vi "Test Data Logger v2 API.vi"() -> ()   [LabVIEW 2025, in "Data Logger v2.lvlib"]
doc: "Data Logger v2 API Tester.\n\n<b>Note:</b> This VI was modified by the <b>Validate DQMH Module</b> tool to upgrade it to the DQMH 5.0 approach to only call the Stop Module.vi at the end of the tester if the module wasn't originally running when the tester started.\n\n<b>Note:</b> This VI was modified by the <b>Validate DQMH Module</b> tool to upgrade its Error Reported event frame to use an improved mechanism for displaying error information.\n\n<b>Note:</b> This VI was modified by the <b>Validate DQMH Module</b> tool to remove code to stop the main loop on error, and instead display the most recent error on the tester front panel."
uses:
  Data Logger v2.lvlib
  Write TDMS 2D Array Parameters--cluster.ctl
  Write TDMS 2D String Array Parameters--cluster.ctl
  <vilib>/Utility/error.llb/DialogType.ctl
  <vilib>/MGI/Panel Manager/Panel/Panel/Window/Window.lvclass
  <vilib>/MGI/Panel Manager/Panel/Panel/Window/Dialog/Dialog.lvclass
  <vilib>/MGI/Panel Manager/Panel/Panel/Subpanel/Subpanel.lvclass
  <vilib>/MGI/Panel Manager/Panel/Panel/Window/Window.vi
  <vilib>/MGI/Panel Manager/Panel/Panel/Window/Dialog/Dialog.vi
  <vilib>/MGI/Panel Manager/Panel/Panel/Subpanel/Subpanel.vi
  <vilib>/MGI/Panel Manager/Panel/Panel.lvlib
panel:
  in  "Property names":string[](array[string])
  in  "Property values":variant[](array[variant])
  in  "Group name":string
  in  "Channel name":string
  in  "Set Properties":bool
  out "last error":errorcluster
  in  "Filename":string
  in  "Create New TDMS Log File (Relative Path)":bool
  in  "Root Folder Path":path
  in  "Set Root Folder Path":bool
  in  "TDMS Write 2D String Array Parameters":T1
  in  "Write TDMS 2D String Array":bool
  in  "Close TDMS File":bool
  in  "TDMS Write 2D Array Parameters":T2
  in  "Write 2D Array to TDMS Log File":bool
  in  "File Path (inc. Filename)":path
  in  "Create New TDMS Log File":bool
  in  "Autoshow?":bool
  in  "Panel Type":enum16{"Window", "Dialog", "Subpanel"}(ring)
  in  "Change Panel":bool
  in  "Tab Control":enum32{"Status", "Subpanel"}(tab)
  out "Status":string
  in  "Show Block Diagram":bool
  in  "Stop Module":bool
  in  "Start Module":bool
  in  "Hide Module Panel":bool
  in  "Show Module Panel":bool
  out "Module Running?":bool
  # "This VI tests the API for the Module."
  # "Change Panel"
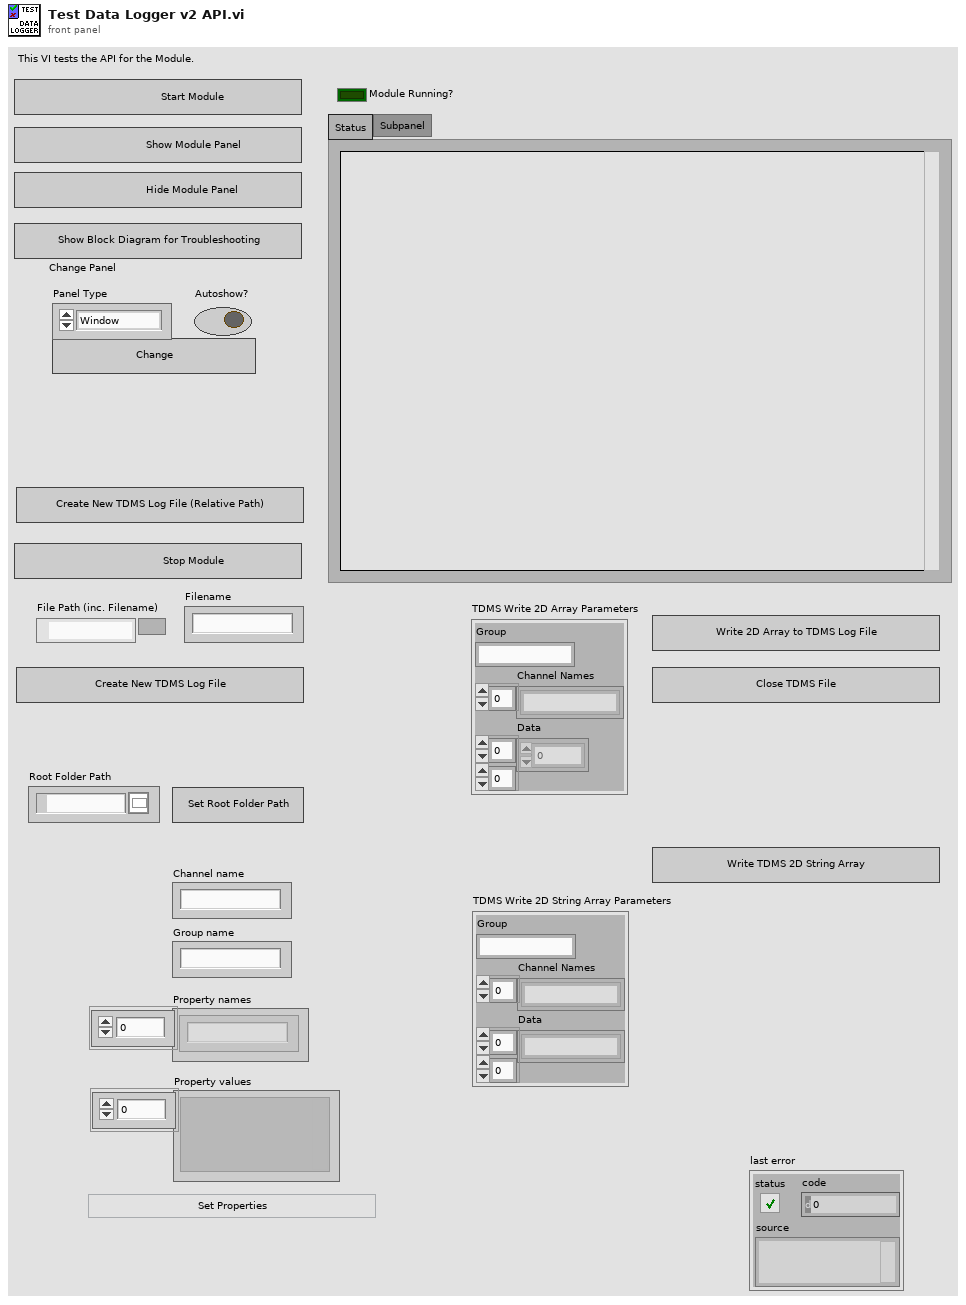
[diagram p1: front panel]
types:
  T1 = typedef "Data Logger v2.lvlib/Write TDMS 2D String Array Parameters--cluster.ctl" = cluster{"Group":string, "Channel Names":string[], "Data":string[][]}
  T2 = typedef "Data Logger v2.lvlib/Write TDMS 2D Array Parameters--cluster.ctl" = cluster{"Group":string, "Channel Names":string[], "Data":dbl[][]}
  T3 = typedef "Data Logger v2.lvlib/Broadcast Events--cluster.ctl" = cluster{"Module Did Init":refnum<user-event>, "Status Updated":refnum<user-event>, "Error Reported":refnum<user-event>, "Module Did Stop":refnum<user-event>, "Update Module Execution Status":refnum<user-event>}
  T4 = typedef "DialogType.ctl" = u16
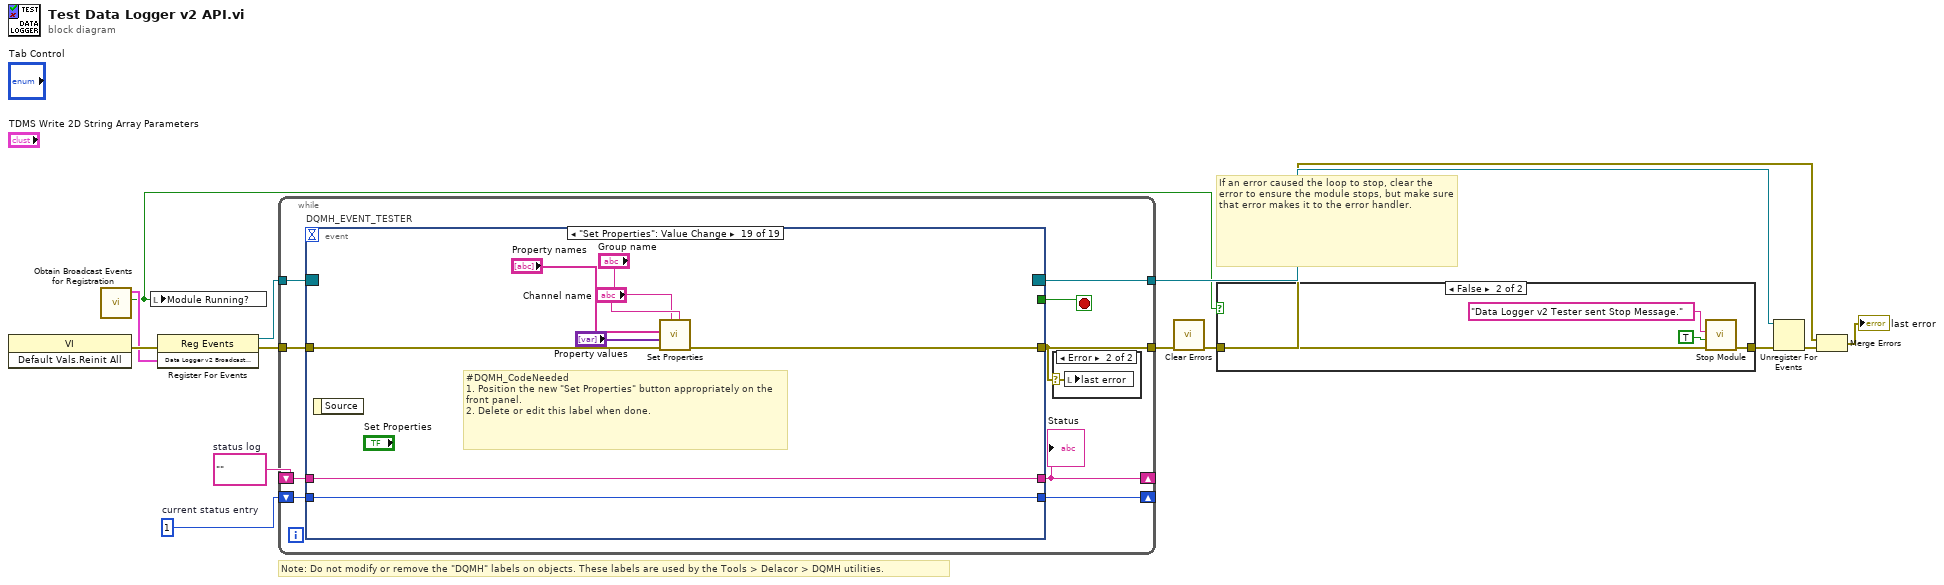
[diagram p0: block diagram]
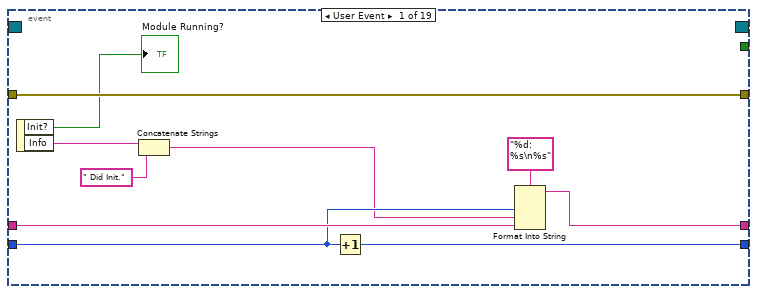
[diagram p4: hidden frame]
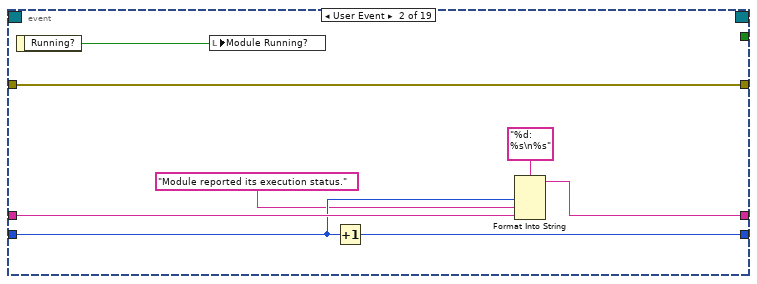
[diagram p5: hidden frame]
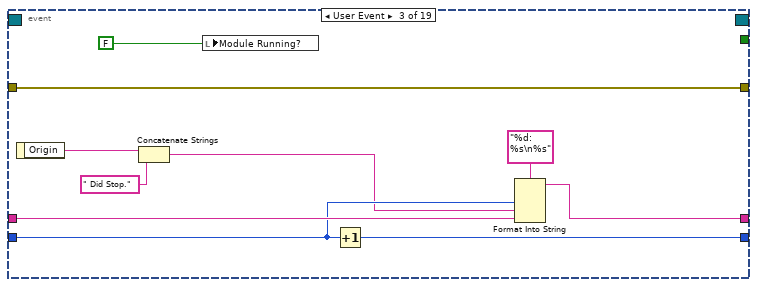
[diagram p6: hidden frame]
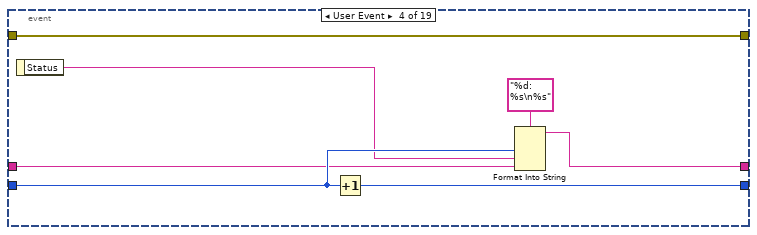
[diagram p7: hidden frame]
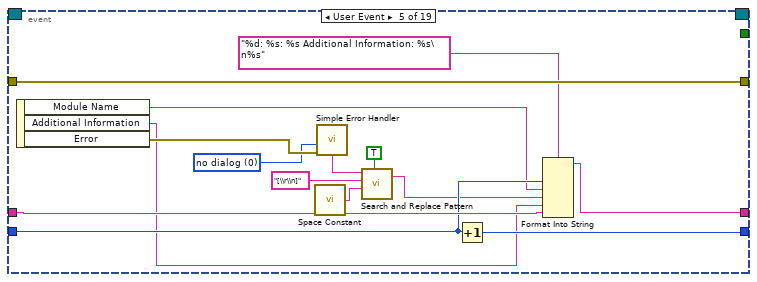
[diagram p8: hidden frame]
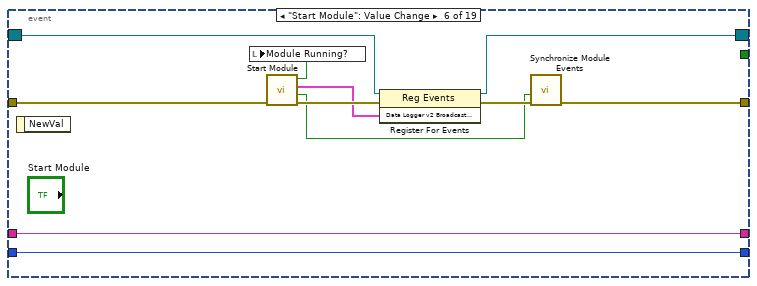
[diagram p9: hidden frame]
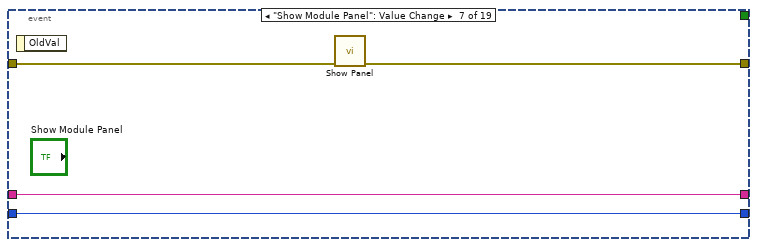
[diagram p10: hidden frame]
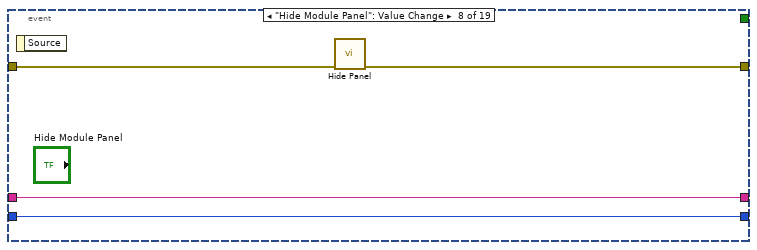
[diagram p11: hidden frame]
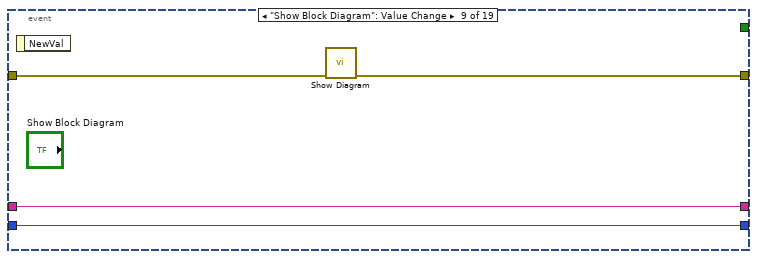
[diagram p12: hidden frame]
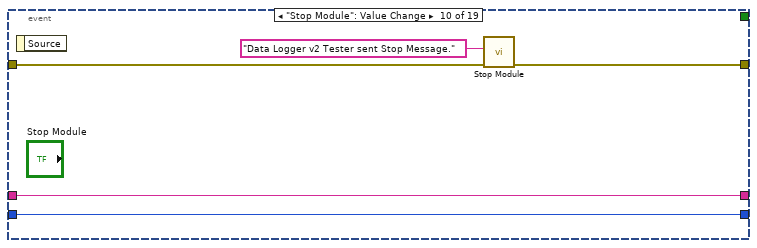
[diagram p13: hidden frame]
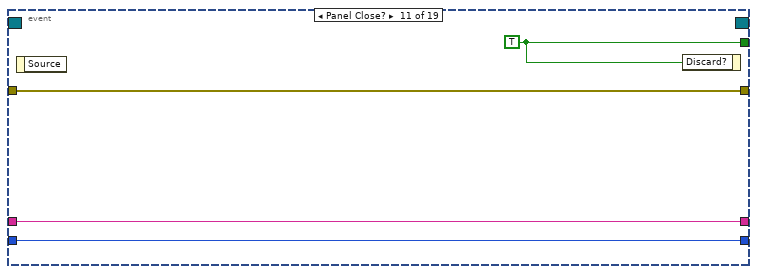
[diagram p14: hidden frame]
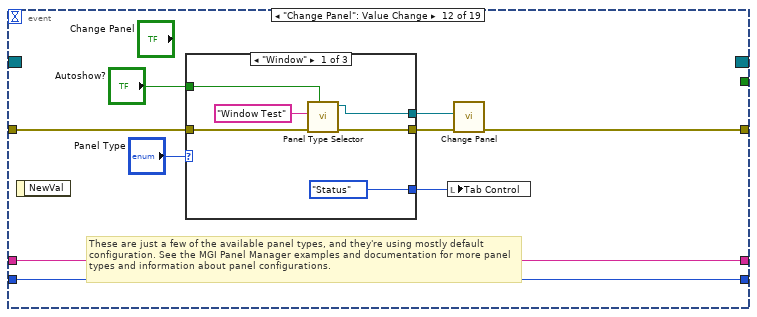
[diagram p15: hidden frame]
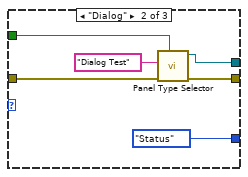
[diagram p16: hidden frame]
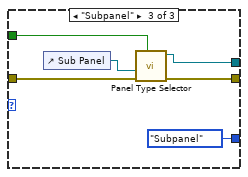
[diagram p17: hidden frame]
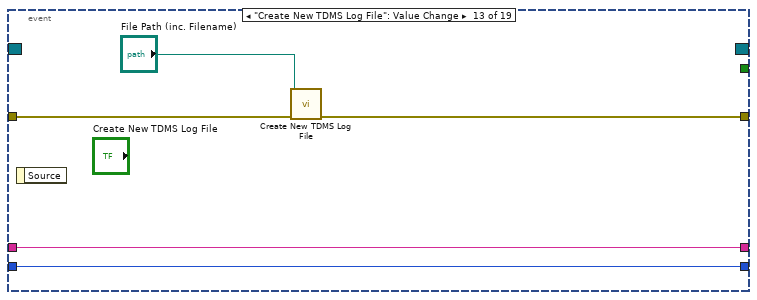
[diagram p18: hidden frame]
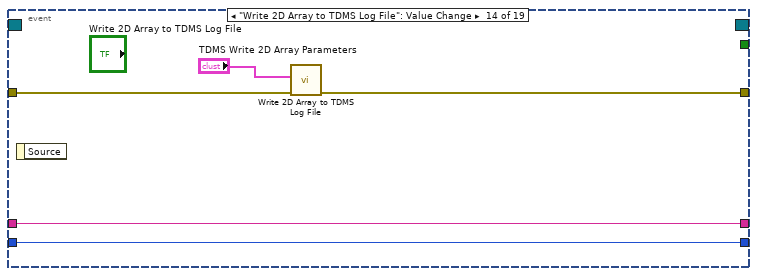
[diagram p19: hidden frame]
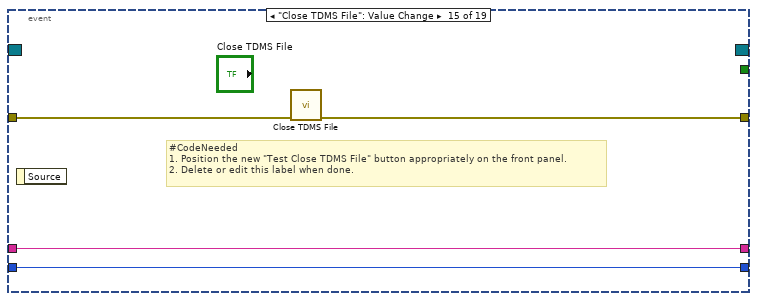
[diagram p20: hidden frame]
diagram:
  w10 = 1  # current status entry
  w11 = ""  # status log
  # "If an error caused the loop to stop, clear the error to ensure the module stops, but make sure that error makes it to the error handler."
  # "Note: Do not modify or remove the \"DQMH\" labels on objects. These labels are used by the Tools > Delacor > DQMH utilities."
  n1 = invoke class="VI" method="Default Vals.Reinit All"() -> (error out=w9:errorcluster)  [unwired: 3 in, 2 out]
  n2 = call "Obtain Broadcast Events for Registration.vi"() -> ("Already running?"=w2:bool, "Data Logger v2 Broadcast Events"=w7:T3)  [unwired: 9 in, 1 out]
  n3 = local write "Module Running?"(w2) -> ()
  n4 = register-events(error in=w9, w7) -> (reference out=w6:refnum<event-registration>, error out=w8:errorcluster)  [unwired: 1 in]
  n5 = while {
    tunnel: w6 -> [w22]
    tunnel: [w15] -> w3
    shift-right: [w18] -> _
    shift-left: w11 -> [w20]
    shift-right: [w19] -> _
    shift-left: w10 -> [w21]
    tunnel: w8 -> [w17]
    tunnel: [w16] -> w5
    stop <- w14 stop-if-true
    n6 = event "DQMH_EVENT_TESTER" shown="[18] \"Set Properties\": Value Change" {
      selector: w22 -> [_ _ _ _ _ w78 _ _ _ _ _ _ _ _ _ _ _ _ _]
      dyn-events: [_ _ _ _ _ w77 _ _ _ _ _ _ _ _ _ _ _ _ _] -> w16
      timeout: _ -> [_ _ _ _ _ _ _ _ _ _ _ _ _ _ _ _ _ _ _]
      tunnel: [_ _ _ _ _ _ _ _ _ _ w105 _ _ _ _ _ _ _ _] -> w14
      tunnel: [w33 w35 w42 w52 w73 w76 w88 w92 w93 w99 w102 w112 w134 w139 w143 w147 w152 w157 w165] -> w15
      tunnel: w21 -> [w29 w39 w49 w55 w70 w81 w86 w90 w94 w100 w103 w113 w135 w140 w144 w148 w153 w158 w166]
      tunnel: w20 -> [w30 w40 w50 w54 w72 w82 w87 w91 w95 w101 w104 w114 w136 w141 w145 w149 w154 w159 w167]
      tunnel: [w27 w37 w47 w56 w71 w82 w87 w91 w95 w101 w104 w114 w136 w141 w145 w149 w154 w159 w167] -> w18
      tunnel: [w28 w38 w48 w58 w69 w81 w86 w90 w94 w100 w103 w113 w135 w140 w144 w148 w153 w158 w166] -> w19
      tunnel: w17 -> [w33 w35 w42 w52 w73 w74 w85 w89 w96 w97 w102 w111 w137 w142 w146 w150 w155 w160 w168]
      event User Event {
        n7 = event-data() -> ("Init?"=→"Module Running?":bool, "Info"=w26:string)  [unwired: 1 in]
        n8 = Concatenate Strings(w26, " Did Init.") -> (w25:string)
        n9 = Increment(x=w29) -> (x+1=w28:i32)
        n10 = Format Into String(format string="%d: %s\n%s", w29, w25, w30) -> (resulting string=w27:string)  [unwired: 2 in, 1 out]
      }
      event User Event {
        n11 = event-data() -> ("Running?"=w34:bool)  [unwired: 1 in]
        n12 = local write "Module Running?"(w34) -> ()
        n13 = Increment(x=w39) -> (x+1=w38:i32)
        n14 = Format Into String(format string="%d: %s\n%s", w39, "Module reported its execution status.", w40) -> (resulting string=w37:string)  [unwired: 2 in, 1 out]
      }
      event User Event {
        n15 = event-data() -> ("Origin"=w46:string)  [unwired: 1 in]
        n16 = Concatenate Strings(w46, " Did Stop.") -> (w45:string)
        n17 = local write "Module Running?"(FALSE ("Module Did Init?")) -> ()
        n18 = Increment(x=w49) -> (x+1=w48:i32)
        n19 = Format Into String(format string="%d: %s\n%s", w49, w45, w50) -> (resulting string=w47:string)  [unwired: 2 in, 1 out]
      }
      event User Event {
        n20 = event-data() -> ("Status"=w53:string)  [unwired: 1 in]
        n21 = Increment(x=w55) -> (x+1=w58:i32)
        n22 = Format Into String(format string="%d: %s\n%s", w55, w53, w54) -> (resulting string=w56:string)  [unwired: 2 in, 1 out]
      }
      event User Event {
        w65 = T4 0 items=["no dialog", "OK message", "continue or stop message", "OK message + warnings", "continue/stop + warnings"] ("type of dialog (OK msg:1)")
        n23 = event-data() -> ("Module Name"=w66:string, "Additional Information"=w67:string, "Error"=w68:errorcluster)  [unwired: 1 in]
        n24 = call <vilib>:"Space Constant.vi"() -> ("String"=w61:string)
        n25 = call <vilib>:"Simple Error Handler.vi"("type of dialog (OK msg:1)"=w65, "error in (no error)"=w68) -> ("message"=w64:string)  [unwired: 3 in, 4 out]
        n26 = call <vilib>:"Search and Replace Pattern.vi"("string"=w64, "regular expression (\"\")"="[\\r\\n]" ("regular expression (\"\")"), "replace string (\"\")"=w61, "replace all? (F)"=TRUE ("replace all CR/LF with spaces")) -> ("result string"=w63:string)  [unwired: 1 in, 1 out]
        n27 = Increment(x=w70) -> (x+1=w69:i32)
        n28 = Format Into String(format string="%d: %s: %s Additional Information: %s\n%s", w70, w66, w63, w67, w72) -> (resulting string=w71:string)  [unwired: 2 in, 1 out]
      }
      event "Start Module": Value Change {
        n29 = event-data() -> ()  [unwired: 1 in, 1 out]
        n30 = call "Start Module.vi"("error in (no error)"=w74) -> ("error out"=w83:errorcluster, "Wait for Event Sync?"=w80:bool, "Data Logger v2 Broadcast Events"=w79:T3, "Module Was Already Running?"=w75:bool)  [unwired: 7 in]
        n31 = local write "Module Running?"(w75) -> ()
        n32 = register-events(reference=w78, error in=w83, w79) -> (reference out=w77:refnum<event-registration>, error out=w84:errorcluster)
        n33 = call "Synchronize Module Events.vi"("error in (no error)"=w84, "Wait for Event Sync?"=w80) -> ("error out"=w76:errorcluster)  [unwired: 9 in]
      }
      event "Show Module Panel": Value Change {
        n34 = event-data() -> ()  [unwired: 1 in, 1 out]
        n35 = call "Show Panel.vi"("error in (no error)"=w85) -> ("error out"=w88:errorcluster)  [unwired: 10 in]
      }
      event "Hide Module Panel": Value Change {
        n36 = event-data() -> ()  [unwired: 1 in, 1 out]
        n37 = call "Hide Panel.vi"("error in (no error)"=w89) -> ("error out"=w92:errorcluster)  [unwired: 10 in]
      }
      event "Show Block Diagram": Value Change {
        n38 = event-data() -> ()  [unwired: 1 in, 1 out]
        n39 = call "Show Diagram.vi"("error in (no error)"=w96) -> ("error out"=w93:errorcluster)  [unwired: 10 in]
      }
      event "Stop Module": Value Change {
        n40 = event-data() -> ()  [unwired: 1 in, 1 out]
        n41 = call "Stop Module.vi"("error in (no error)"=w97, "Origin"="Data Logger v2 Tester sent Stop Message.") -> ("error out"=w99:errorcluster)  [unwired: 9 in]
      }
      event Panel Close? {
        w105 = TRUE ("Discard?")
        n42 = event-data() -> ()  [unwired: 1 in, 1 out]
        n43 = event-data("Discard?"=w105) -> ()  [unwired: 1 in, 1 out]
      }
      event "Change Panel": Value Change {
        # "These are just a few of the available panel types, and they're using mostly default configuration. See the MGI Panel Manager examples and documentation for more panel types and information about panel configurations."
        n44 = event-data() -> ()  [unwired: 1 in, 1 out]
        n45 = case shown="\"Window\"" "Panel Type" {
          tunnel: w111 -> [w120 w126 w132]
          tunnel: [w119 w125 w131] -> w110
          tunnel: [w118 w124 w130] -> w109
          tunnel: [enum32{"Status", "Subpanel"}."Status" ("Tab Control") enum32{"Status", "Subpanel"}."Status" ("Tab Control") enum32{"Status", "Subpanel"}."Subpanel" ("Tab Control")] -> w107
          tunnel: "Autoshow?" -> [w115 w121 w127]
          frame "Window" {
            n46 = call-poly <vilib>:"Panel Type Selector.vi"("Autoshow? (T)"=w115, "error in (no error)"=w120, "Default Title"="Window Test") -> ("error out"=w119:errorcluster, "Window out"=w118:refnum<class "Window.lvclass">)  [unwired: 7 in]
          }
          frame "Dialog" {
            n47 = call-poly <vilib>:"Panel Type Selector.vi"("Autoshow? (T)"=w121, "Error In"=w126, "Default Title"="Dialog Test") -> ("Error Out"=w125:errorcluster, "Dialog out"=w124:refnum<class "Dialog.lvclass">)  [unwired: 7 in]
          }
          frame "Subpanel" {
            n48 = control-ref of="Sub Panel"() -> (w129:refnum<vi>)
            n49 = call-poly <vilib>:"Panel Type Selector.vi"("Autoshow? (T)"=w127, "Error In"=w132, "Sub Panel"=w129) -> ("Error Out"=w131:errorcluster, "Subpanel Out"=w130:refnum<class "Subpanel.lvclass">)  [unwired: 7 in]
          }
        }
        n50 = local write "Tab Control"(w107) -> ()
        n51 = call "Change Panel.vi"("error in (no error)"=w110, "New Panel"=w109) -> ("error out"=w112:errorcluster)  [unwired: 9 in]
      }
      event "Create New TDMS Log File": Value Change {
        n52 = event-data() -> ()  [unwired: 1 in, 1 out]
        n53 = call "Create New TDMS Log File.vi"("error in (no error)"=w137, "File Path (inc. Filename)"="File Path (inc. Filename)") -> ("error out"=w134:errorcluster)  [unwired: 9 in]
      }
      event "Write 2D Array to TDMS Log File": Value Change {
        n54 = event-data() -> ()  [unwired: 1 in, 1 out]
        n55 = call "Write 2D Array to TDMS Log File.vi"("error in (no error)"=w142, "TDMS Write 2D Array Parameters"="TDMS Write 2D Array Parameters") -> ("error out"=w139:errorcluster)  [unwired: 9 in]
      }
      event "Close TDMS File": Value Change {
        # "#CodeNeeded\n1. Position the new \"Test Close TDMS File\" button appropriately on the front panel.\n2. Delete or edit this label when done."
        n56 = event-data() -> ()  [unwired: 1 in, 1 out]
        n57 = call "Close TDMS File.vi"("error in (no error)"=w146) -> ("error out"=w143:errorcluster)  [unwired: 10 in]
      }
      event "Write TDMS 2D String Array": Value Change {
        # "#CodeNeeded\n1. Position the new \"Test Write TDMS 2D String Array\" button appropriately on the front panel.\n2. Delete or edit this label when done."
        n58 = event-data() -> ()  [unwired: 1 in, 1 out]
        n59 = call "Write TDMS 2D String Array.vi"("error in (no error)"=w150) -> ("error out"=w147:errorcluster)  [unwired: 10 in]
      }
      event "Set Root Folder Path": Value Change {
        # "#CodeNeeded\n1. Position the new \"Test Set Root Folder Path\" button appropriately on the front panel.\n2. Delete or edit this label when done."
        n60 = event-data() -> ()  [unwired: 1 in, 1 out]
        n61 = call "Set Root Folder Path.vi"("error in (no error)"=w155, "Root Folder Path"="Root Folder Path") -> ("error out"=w152:errorcluster)  [unwired: 9 in]
      }
      event "Create New TDMS Log File (Relative Path)": Value Change {
        # "#CodeNeeded\n1. Position the new \"Test Create New TDMS Log File (Relative Path)\" button appropriately on the front panel.\n2. Delete or edit this label when done."
        n62 = event-data() -> ()  [unwired: 1 in, 1 out]
        n63 = call "Create New TDMS Log File (Relative Path).vi"("error in (no error)"=w160, "Filename"="Filename") -> ("error out"=w157:errorcluster)  [unwired: 9 in]
      }
      event "Set Properties": Value Change {
        # "#DQMH_CodeNeeded\n1. Position the new \"Set Properties\" button appropriately on the front panel.\n2. Delete or edit this label when done."
        n64 = event-data() -> ()  [unwired: 1 in, 1 out]
        n65 = call "Set Properties.vi"("Group name"="Channel name", "Channel name"="Group name", "error in"=w168, "Property values"="Property values", "Property names"="Property names") -> ("error out"=w165:errorcluster)  [unwired: 6 in]
      }
    }
    "Status" <- w18
    n66 = case "DQMH_TESTER_ERROR_LOCAL" shown="Error" w15 {
      selector: w15 -> [_ w23]
      frame No Error {
      }
      frame Error {
        n67 = local write "last error"(w23) -> ()
      }
    }
  }
  n68 = call <vilib>:"Clear Errors.vi"("error in (no error)"=w3) -> ("error out"=w4:errorcluster)  [unwired: 5 in, 1 out]
  n69 = case shown="False" w2 {
    tunnel: [w169 w173] -> w12
    tunnel: w4 -> [w169 w170]
    frame True {
    }
    frame False {
      n70 = call "Stop Module.vi"("error in (no error)"=w170, "Wait for Module to Stop? (F)"=TRUE ("Wait for Module to stop?"), "Origin"="Data Logger v2 Tester sent Stop Message.") -> ("error out"=w173:errorcluster)  [unwired: 8 in]
    }
  }
  n71 = Unregister For Events(event registration refnum=w5, error in=w12) -> (error out=w13:errorcluster)
  n72 = Merge Errors(w3, w13) -> (→"last error":errorcluster)
